vi "datasource.from_json.vi"(8 "error in":errorcluster, 10 "json":string) -> (0 "error out":errorcluster, 2 "dataSource":T1)   [LabVIEW 2020, in "dataScopes.lvlib"]
uses:
  dataScopes.lvlib
  7d87e695-0c51-4d0d-8beb-747f1085477c.vi
  <vilib>/JDP Science/JSONtext/Next JSON Value.vi
  <vilib>/JDP Science/JSONtext/String Subset.vi
  <vilib>/JDP Science/JSONtext/Parsing/Advance past next JSON Value (inlined COPY).vi
  <vilib>/JDP Science/JSONtext/Parsing/Advance past whitespace.vi
  <vilib>/JDP Science/JSONtext/Parsing/Advance past String.vi
  <vilib>/JDP Science/JSONtext/Parsing/Advance past Number.vi
  <vilib>/JDP Science/JSONtext/Parsing/Advance past Line Ending.vi
  <vilib>/JDP Science/JSONtext/Parsing/Parse Full Path or Item Name.vi
  <vilib>/JDP Science/JSONtext/Parsing/Advance past Array.vi
  <vilib>/JDP Science/JSONtext/Parsing/Advance past Object.vi
  <vilib>/JDP Science/JSONtext/support/Error Cluster From Code.vi
  <vilib>/JDP Science/JSONtext/Offset/Find Item Locations by Path.vi
  <vilib>/JDP Science/JSONtext/JSON text to Variant.vi
  <vilib>/JDP Science/JSONtext/LVClass Serializer/JSONtext LVClass Serializer.lvclass
  <vilib>/JDP Science/JSONtext/JSONtext.lvlib
  e5b7be2a-dd82-4e76-91a8-ac3345dfd91b.vi
  type.ctl
  data_source.ctl
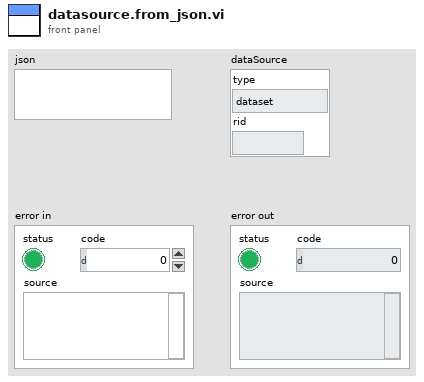
[diagram p1: front panel]
types:
  T1 = typedef "dataScopes.lvlib/data_source.ctl" = cluster{"type":T2, "rid":string}
  T2 = typedef "dataScopes.lvlib/type.ctl" = enum16{"dataset", "connection", "logSet", "video"}
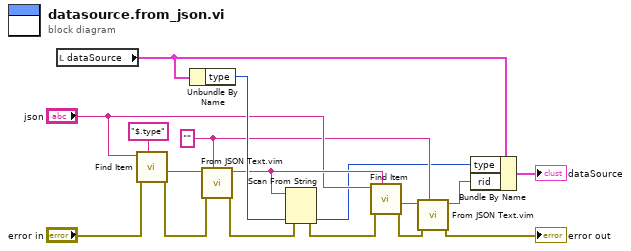
[diagram p0: block diagram]
diagram:
  w7 = "" ("$Path or Item Name")
  n1 = local read "dataSource"() -> (w1:T1)
  n2 = call <vilib>:"Find Item.vi"("$Path or Item Name"="$.type", "error in (no error)"="error in", "JSON"="json") -> ("error out"=w13:errorcluster, "<JSON>"=w15:string)  [unwired: 5 in, 2 out]
  n3 = Unbundle By Name(w1) -> ("type"=w16:T2)
  n4 = call "From JSON Text.vim"("Data Type and Default Value"=w7, "error in (no error)"=w13, "JSON"=w15) -> ("error out"=w14:errorcluster, "Data out"=w11:string)  [unwired: 7 in]
  n5 = Scan From String(input string=w11, error in=w14, default 1=w16) -> (error out=w6:errorcluster, output 1=w3:T2)  [unwired: 2 in, 2 out]
  n6 = call <vilib>:"Find Item.vi"("$Path or Item Name"=w11, "error in (no error)"=w6, "JSON"="json") -> ("error out"=w8:errorcluster, "<JSON>"=w9:string)  [unwired: 5 in, 2 out]
  n7 = call "From JSON Text.vim"("Data Type and Default Value"=w7, "error in (no error)"=w8, "JSON"=w9) -> ("error out"=→"error out":errorcluster, "Data out"=w2:string)  [unwired: 7 in]
  n8 = Bundle By Name(cluster=w1, "type"=w3, "rid"=w2) -> (→"dataSource":T1)
